vi "ProcessHandshakeRequest.vi"(0 "HTTP Headers":string, 11 "error in (no error)":errorcluster) -> (3 "Host":string, 4 "Is Websocket Request?":bool, 6 "URI":string, 8 "Resource Name":string, 10 "Sec-WebSocket-Key":string, 14 "Headers Out":variant, 15 "error out":errorcluster)   [LabVIEW 2016, in "WebSockets.lvlib"]
doc: "Converts the raw HTTP header string into it's main component parts needed to check if the incoming connection is a WS connection. The additional headers are returned in a variant lookup table.\nWebSockets 1.6.0.22\nSam Sharp - MediaMongrels Ltd\nCopyright (c) 2016, MediaMongrels Ltd"
uses:
  WebSockets.lvlib
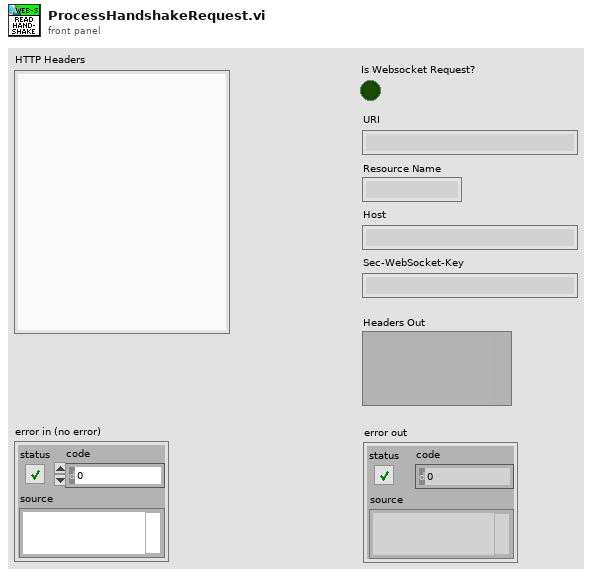
[diagram p1: front panel]
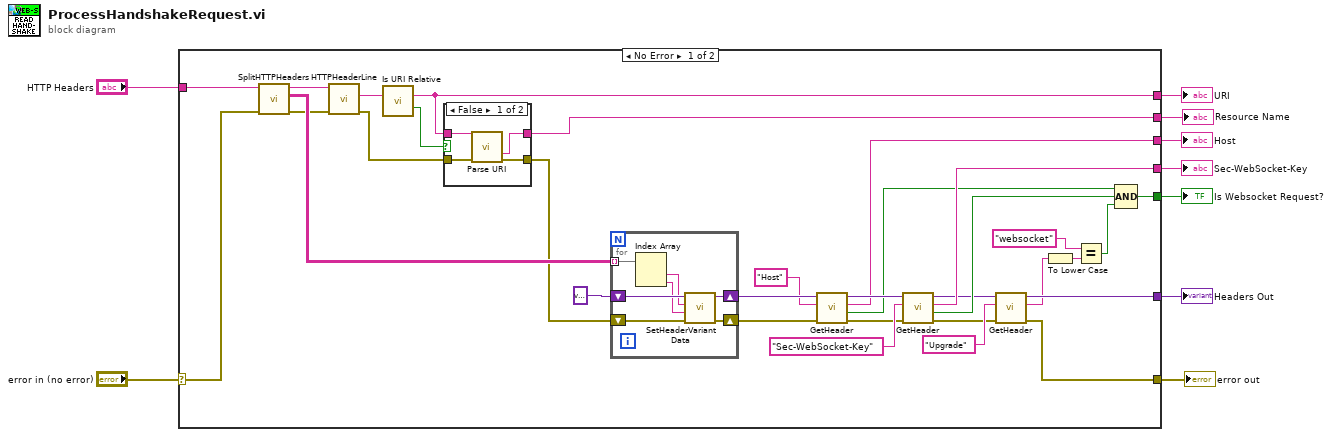
[diagram p0: block diagram]
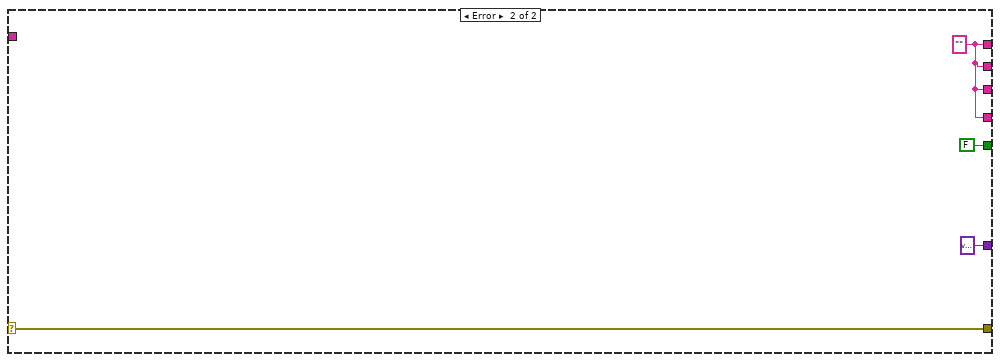
[diagram p3: hidden frame]
diagram:
  n1 = case shown="No Error" "error in (no error)" {
    selector: "error in (no error)" -> [w23 w58]
    tunnel: "HTTP Headers" -> [w41 _]
    tunnel: [w13 w55] -> w8
    tunnel: [w34 w55] -> w7
    tunnel: [w32 w55] -> w6
    tunnel: [w28 variant ("Headers Out")] -> w5
    tunnel: [w24 FALSE] -> w4
    tunnel: [w19 w58] -> w2
    tunnel: [w12 w55] -> w1
    frame No Error {
      n2 = call "SplitHTTPHeaders.vi"("error in (no error)"=w23, "HTTP Header String"=w41) -> ("error out"=w22:errorcluster, "Headers Array"=w39:string[][], "HTTP Request"=w40:string)  [unwired: 7 in]
      n3 = call "HTTPHeaderLine.vi"("error in (no error)"=w22, "HTTP Request Line"=w40) -> ("error out"=w11:errorcluster, "Request URI"=w15:string)  [unwired: 6 in, 2 out]
      n4 = call "Is URI Relative.vi"("URI"=w15) -> ("URI Out"=w13:string, "Relative"=w14:bool)  [unwired: 13 in]
      n5 = case shown="False" w14 {
        tunnel: w13 -> [w45 w47]
        tunnel: [w43 w47] -> w12
        tunnel: w11 -> [w44 w46]
        tunnel: [w42 w46] -> w10
        frame False {
          n6 = call "Parse URI.vi"("URI"=w45, "error in"=w44) -> ("Resource Name"=w43:string, "error out"=w42:errorcluster)  [unwired: 8 in, 4 out]
        }
        frame True {
        }
      }
      n7 = for {
        tunnel: w39 -> [w54] mode=indexing
        shift-right: [w53] -> w37
        shift-left: variant -> [w50]
        shift-right: [w52] -> w18
        shift-left: w10 -> [w51]
        n8 = Index Array(array=w54) -> (element #1=w49:string, element #2=w48:string)  [unwired: 2 in]
        n9 = call "SetHeaderVariantData.vi"("error in (no error)"=w51, "Value"=w48, "Name"=w49, "Variant in"=w50) -> ("error out"=w52:errorcluster, "Variant out"=w53:variant)  [unwired: 6 in]
      }
      n10 = call "GetHeader.vi"("error in (no error)"=w18, "Name"="Host" ("name"), "Headers In"=w37) -> ("error out"=w21:errorcluster, "Found?"=w31:bool, "Data"=w34:string, "Headers Out"=w35:variant)  [unwired: 5 in]
      n11 = call "GetHeader.vi"("error in (no error)"=w21, "Name"="Sec-WebSocket-Key", "Headers In"=w35) -> ("error out"=w20:errorcluster, "Found?"=w30:bool, "Data"=w32:string, "Headers Out"=w29:variant)  [unwired: 5 in]
      n12 = call "GetHeader.vi"("error in (no error)"=w20, "Name"="Upgrade", "Headers In"=w29) -> ("error out"=w19:errorcluster, "Data"=w17:string, "Headers Out"=w28:variant)  [unwired: 5 in, 1 out]
      n13 = To Lower Case(string=w17) -> (all lower case string=w16:string)
      n14 = Equal?(x="websocket", y=w16) -> (x = y?=w25:bool)
      n15 = Compound Arithmetic op=AND(w31, w30, w25) -> (w24:bool)
    }
    frame Error {
      w55 = "" ("Request URI")
    }
  }
  "Host" <- w7
  "URI" <- w8
  "Sec-WebSocket-Key" <- w6
  "Is Websocket Request?" <- w4
  "Headers Out" <- w5
  "error out" <- w2
  "Resource Name" <- w1
